vi "openDocument.vi"(8 "error in (no error)":errorcluster, 11 "workbook in":refnum<class "workbook.lvclass">) -> (0 "error out":errorcluster, 3 "workbook out":refnum<class "workbook.lvclass">)   [LabVIEW 2017, in "Excel_Specific.lvlib" / "workbook.lvclass"]
uses:
  workbook.lvclass
  C:/Users/Neo/Desktop/Dev_Tools_BR/LabVIEW_NPOI/src/LabVIEW NPOI/NPOI_Document/npoiDocument/npoiDocument.lvclass
  NPOI_Document/npoiDocument/npoiDocument.lvclass/npoiDocument.ctl
  C:/Users/Neo/Desktop/Dev_Tools_BR/LabVIEW_NPOI/src/lib/NPOI 2.1.1/NPOI.OOXML.dll
  lib/NPOI 2.1.1/NPOI.OOXML.dll
  workbook.lvclass/workbook.ctl
  NPOI_Document/npoiDocument/Get Document.Path.vi
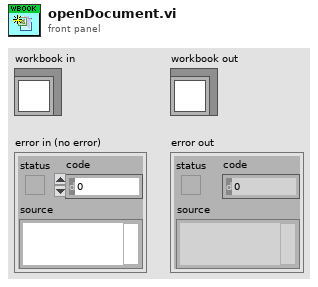
[diagram p1: front panel]
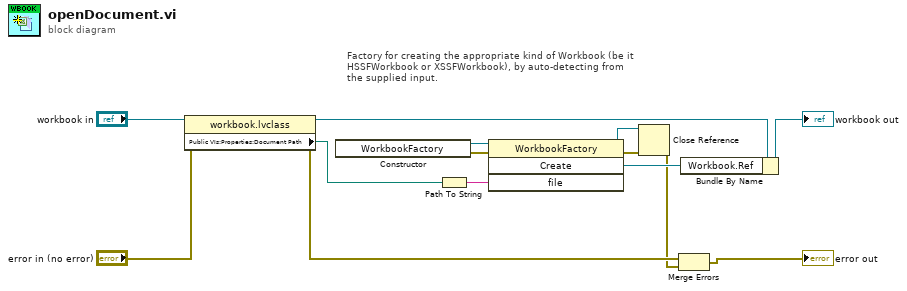
[diagram p0: block diagram]
diagram:
  # "Factory for creating the appropriate kind of Workbook (be it HSSFWorkbook or XSSFWorkbook), by auto-detecting from the supplied input."
  n1 = property class="workbook.lvclass"(reference="workbook in", error in="error in (no error)") -> (reference out=w6:refnum<class "workbook.lvclass">, error out=w3:errorcluster, "Public VIs:Properties:Document Path"=w9:path)
  n2 = constructor class="WorkbookFactory"() -> (reference out=w14:refnum<k24>, error out=w13:errorcluster)  [unwired: 3 in, 1 out]
  n3 = Path To String(path=w9) -> (string=w8:string)
  n4 = invoke class="WorkbookFactory" method="Create"(reference=w14, error in=w13, "file"=w8) -> (reference out=w12:refnum<k24>, error out=w10:errorcluster, "Create"=w11:refnum<k24>)  [unwired: 1 in, 1 out]
  n5 = Close Reference(reference=w12, error in (no error)=w10) -> (error out=w1:errorcluster)
  n6 = Merge Errors(w3, w1) -> (→"error out":errorcluster)
  n7 = Bundle By Name(cluster=w6, "Workbook.Ref"=w11) -> (→"workbook out":refnum<class "workbook.lvclass">)
